vi "Funct TIFF export-Custom Write multi-page TIFF.vi"(6 "Image Pixels (U16)":u16[][](array[numeric]), 7 "totalpages":i32, 8 "error in (no error)":errorcluster, 9 "page":u32, 11 "Handle":i32) -> (0 "error out":errorcluster, 3 "Handle out":i32)   [LabVIEW 2017]
doc: "SciScan 1.0 151216\nWrite a U16 page using LIBTIFFwriteEncodedStrip to a file previously open for writing"
uses:
  support/Libtiff3/DLLs/libtiff3 (32).dll
panel:
  out "status_compression":i32
  out "status width":i32
  out "status_length":i32
  out "status_spp":i32
  out "status_bps":i32
  out "status_orientation":i32
  out "status_planarconfig":i32
  out "status_photo":i32
  out "status_rowperstrip":i32
  out "status_writeencodestrip":i32
  out "status_subfile":i32
  out "status_writedir":i32
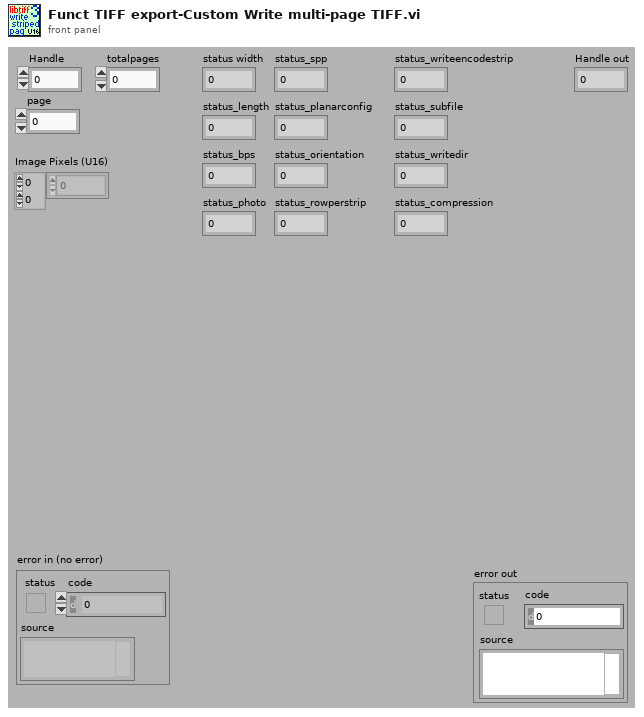
[diagram p1: front panel]
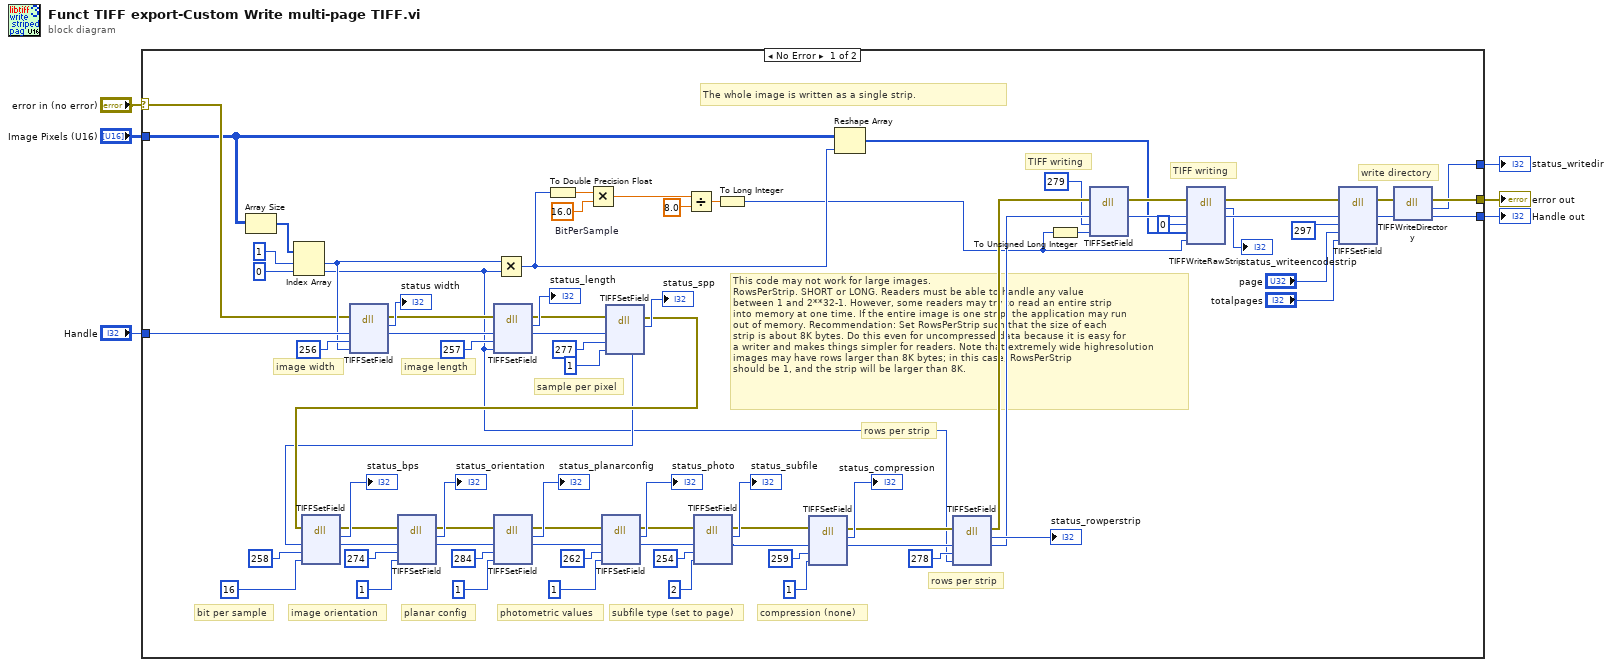
[diagram p0: block diagram]
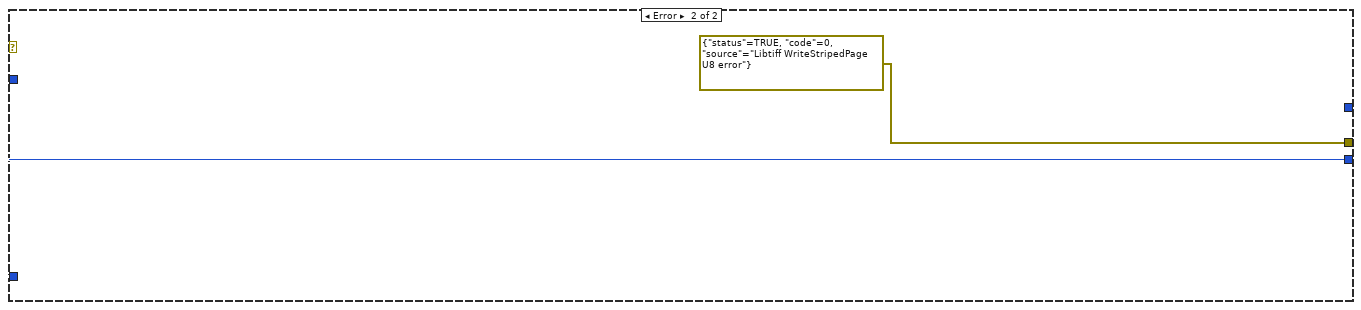
[diagram p2: hidden frame]
diagram:
  n1 = case shown="No Error" "error in (no error)" {
    selector: "error in (no error)" -> [w19 _]
    tunnel: "Handle" -> [w58 w87]
    tunnel: [w54 w87] -> w5
    tunnel: [w41 errorcluster {"status"=TRUE, "code"=0, "source"="Libtiff WriteStripedPage U8 error"} ("error out")] -> w4
    tunnel: [w15 _] -> w2
    tunnel: "Image Pixels (U16)" -> [w18 _]
    frame No Error {
      w24 = 16.0  # BitPerSample
      # "This code may not work for large images.\nRowsPerStrip. SHORT or LONG. Readers must be able to handle any value\nbetween 1 and 2**32-1. However, some readers may try to read an entire strip\ninto memory at one time. If the entire image is one strip, the application may run\nout of memory. Recommendation: Set RowsPerStrip such that the size of each\nstrip is about 8K bytes. Do this even for uncompressed data because it is easy for\na writer and makes things simpler for readers. Note that extremely wide highresolution\nimages may have rows larger than 8K bytes; in this case, RowsPerStrip\nshould be 1, and the strip will be larger than 8K."
      # "TIFF writing"
      # "The whole image is written as a single strip."
      # "TIFF writing"
      # "rows per strip"
      # "rows per strip"
      # "compression (none)"
      # "write directory"
      # "subfile type (set to page)"
      # "photometric values"
      # "planar config"
      # "image orientation"
      # "bit per sample"
      # "sample per pixel"
      # "image length"
      # "image width"
      n2 = Array Size(array=w18) -> (size(s)=w55:i32[])
      n3 = Index Array(array=w55, index #1=1 ("index"), index #2=0 ("index")) -> (element #1=w26:i32, element #2=w16:i32)
      n4 = dll-call lib="C:/Users/ucbtspu/OneDrive - University College London/Local SCC/SilverLab-Microscope-R3-LV2013/support/Libtiff3/DLLs/libtiff3 (32).dll" fn="TIFFSetField"(error in=w19, "Handle"=w58, "TIFF_tag"=256, "Value"=w26) -> (error out=w49:errorcluster, "return type"=→"status width":i32, "Handle"=w83:i32)  [unwired: 4 in, 1 out]
      n5 = dll-call lib="C:/Users/ucbtspu/OneDrive - University College London/Local SCC/SilverLab-Microscope-R3-LV2013/support/Libtiff3/DLLs/libtiff3 (32).dll" fn="TIFFSetField"(error in=w49, "Handle"=w83, "TIFF_tag"=257, "value"=w16) -> (error out=w48:errorcluster, "return type"=→"status_length":i32, "Handle"=w80:i32)  [unwired: 4 in, 1 out]
      n6 = Multiply(x=w26, y=w16) -> (x*y=w20:i32)
      n7 = To Double Precision Float(number=w20) -> (double precision float=w25:dbl)
      n8 = Multiply(x=w25, y=w24) -> (x*y=w23:dbl)
      n9 = dll-call lib="C:/Users/ucbtspu/OneDrive - University College London/Local SCC/SilverLab-Microscope-R3-LV2013/support/Libtiff3/DLLs/libtiff3 (32).dll" fn="TIFFSetField"(error in=w48, "Handle"=w80, "TIFF_tag"=277, "value"=u32 1) -> (error out=w47:errorcluster, "return type"=→"status_spp":i32, "Handle"=w17:i32)  [unwired: 4 in, 1 out]
      n10 = dll-call lib="C:/Users/ucbtspu/OneDrive - University College London/Local SCC/SilverLab-Microscope-R3-LV2013/support/Libtiff3/DLLs/libtiff3 (32).dll" fn="TIFFSetField"(error in=w47, "Handle"=w17, "TIFF_tag"=258, "value"=u32 16) -> (error out=w46:errorcluster, "return type"=→"status_bps":i32, "Handle"=w75:i32)  [unwired: 4 in, 1 out]
      n11 = dll-call lib="C:/Users/ucbtspu/OneDrive - University College London/Local SCC/SilverLab-Microscope-R3-LV2013/support/Libtiff3/DLLs/libtiff3 (32).dll" fn="TIFFSetField"(error in=w46, "Handle"=w75, "TIFF_tag"=274, "value"=u32 1) -> (error out=w45:errorcluster, "return type"=→"status_orientation":i32, "Handle"=w71:i32)  [unwired: 4 in, 1 out]
      n12 = dll-call lib="C:/Users/ucbtspu/OneDrive - University College London/Local SCC/SilverLab-Microscope-R3-LV2013/support/Libtiff3/DLLs/libtiff3 (32).dll" fn="TIFFSetField"(error in=w45, "Handle"=w71, "TIFF_tag"=284, "value"=u32 1) -> (error out=w44:errorcluster, "return type"=→"status_planarconfig":i32, "Handle"=w67:i32)  [unwired: 4 in, 1 out]
      n13 = dll-call lib="C:/Users/ucbtspu/OneDrive - University College London/Local SCC/SilverLab-Microscope-R3-LV2013/support/Libtiff3/DLLs/libtiff3 (32).dll" fn="TIFFSetField"(error in=w44, "Handle"=w67, "TIFF_tag"=262, "value"=u32 1) -> (error out=w43:errorcluster, "return type"=→"status_photo":i32, "Handle"=w62:i32)  [unwired: 4 in, 1 out]
      n14 = Divide(x=w23, y=8.0) -> (x/y=w21:dbl)
      n15 = dll-call lib="C:/Users/ucbtspu/OneDrive - University College London/Local SCC/SilverLab-Microscope-R3-LV2013/support/Libtiff3/DLLs/libtiff3 (32).dll" fn="TIFFSetField"(error in=w43, "Handle"=w62, "TIFF_tag"=254, "value"=u32 2) -> (error out=w42:errorcluster, "return type"=→"status_subfile":i32, "Handle"=w51:i32)  [unwired: 4 in, 1 out]
      n16 = To Long Integer(number=w21) -> (32bit integer=w9:i32)
      n17 = dll-call lib="C:/Users/ucbtspu/OneDrive - University College London/Local SCC/SilverLab-Microscope-R3-LV2013/support/Libtiff3/DLLs/libtiff3 (32).dll" fn="TIFFSetField"(error in=w42, "Handle"=w51, "TIFF_tag"=259, "value"=u32 1) -> (error out=w35:errorcluster, "return type"=→"status_compression":i32, "Handle"=w34:i32)  [unwired: 4 in, 1 out]
      n18 = Reshape Array(w18, w20) -> (w10:u16[])
      n19 = dll-call lib="C:/Users/ucbtspu/OneDrive - University College London/Local SCC/SilverLab-Microscope-R3-LV2013/support/Libtiff3/DLLs/libtiff3 (32).dll" fn="TIFFSetField"(error in=w35, "Handle"=w34, "TIFF_tag"=278, "value"=w16) -> (error out=w36:errorcluster, "return type"=→"status_rowperstrip":i32, "Handle"=w37:i32)  [unwired: 4 in, 1 out]
      n20 = To Unsigned Long Integer(number=w9) -> (unsigned 32bit integer=w7:u32)
      n21 = dll-call lib="C:/Users/ucbtspu/OneDrive - University College London/Local SCC/SilverLab-Microscope-R3-LV2013/support/Libtiff3/DLLs/libtiff3 (32).dll" fn="TIFFSetField"(error in=w36, "Handle"=w37, "TIFF_tag"=279, "value"=w7) -> (error out=w13:errorcluster, "Handle"=w12:i32)  [unwired: 4 in, 2 out]
      n22 = dll-call lib="C:/Users/ucbtspu/OneDrive - University College London/Local SCC/SilverLab-Microscope-R3-LV2013/support/Libtiff3/DLLs/libtiff3 (32).dll" fn="TIFFWriteRawStrip"(error in=w13, "Handle"=w12, "strip"=0, "buffer"=w10, "length"=w9) -> (error out=w33:errorcluster, "return type"=→"status_writeencodestrip":i32, "Handle"=w32:i32)  [unwired: 5 in, 1 out]
      n23 = dll-call lib="C:/Users/ucbtspu/OneDrive - University College London/Local SCC/SilverLab-Microscope-R3-LV2013/support/Libtiff3/DLLs/libtiff3 (32).dll" fn="TIFFSetField"(error in=w33, "Handle"=w32, "TIFF_tag"=297, "page"="page", "totalpages"="totalpages") -> (error out=w27:errorcluster, "Handle"=w31:i32)  [unwired: 5 in, 2 out]
      n24 = dll-call lib="C:/Users/ucbtspu/OneDrive - University College London/Local SCC/SilverLab-Microscope-R3-LV2013/support/Libtiff3/DLLs/libtiff3 (32).dll" fn="TIFFWriteDirectory"(error in=w27, "Handle"=w31) -> (error out=w41:errorcluster, "return type"=w15:i32, "Handle"=w54:i32)  [unwired: 2 in, 1 out]
    }
    frame Error {
    }
  }
  "Handle out" <- w5
  "error out" <- w4
  "status_writedir" <- w2
